vi "2D Table get 1D Rows.vi"(5 "data":string[][](array[string])) -> (2 "Rows":string[](array[string]))   [LabVIEW 2014]
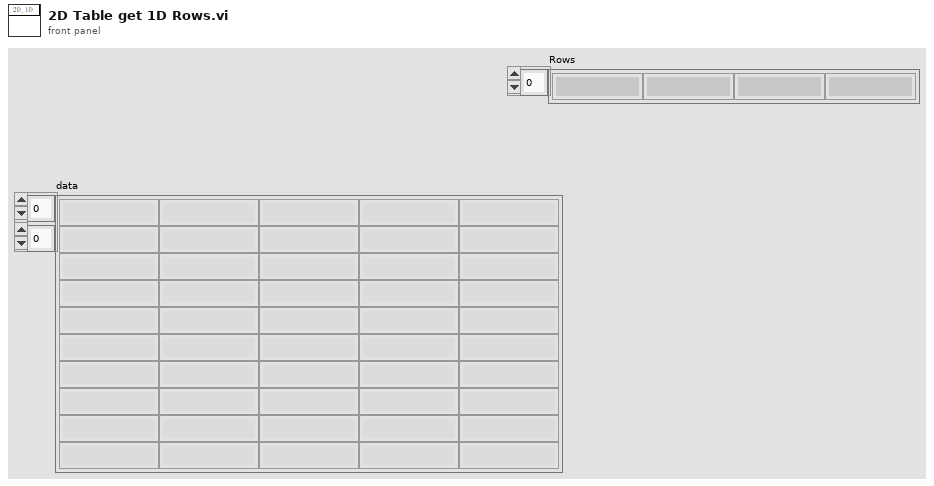
[diagram p1: front panel]
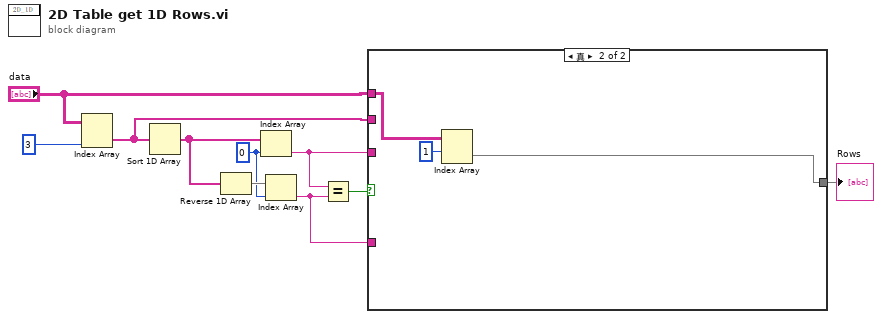
[diagram p0: block diagram]
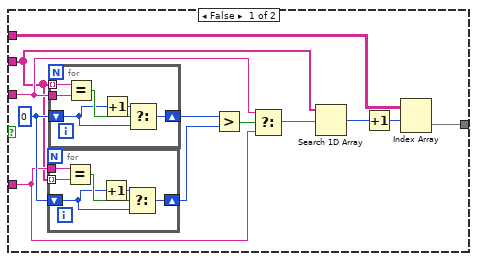
[diagram p2: hidden frame]
diagram:
  w7 = 0 ("index")
  n1 = Index Array(array="data", index (col)=3 ("disabled index (col)")) -> (element=w2:string[])  [unwired: 1 in]
  n2 = Sort 1D Array(array=w2) -> (sorted array=w9:string[])
  n3 = Reverse 1D Array(array=w9) -> (reversed array=w8:string[])
  n4 = Index Array(array=w9, index=w7) -> (element=w4:string)
  n5 = Index Array(array=w8, index=w7) -> (element=w3:string)
  n6 = Equal?(x=w4, y=w3) -> (x = y?=w6:bool)
  n7 = case shown="真" w6 {
    tunnel: "data" -> [w14 w37]
    tunnel: w4 -> [w18 _]
    tunnel: w3 -> [w17 _]
    tunnel: w2 -> [w16 _]
    tunnel: [w13 w35] -> w1
    frame False {
      w22 = 0
      n8 = for {
        tunnel: w16 -> [w28] mode=indexing
        tunnel: w17 -> [w27]
        shift-right: [w26] -> w21
        shift-left: w22 -> [w23]
        n9 = Equal?(x=w27, y=w28) -> (x = y?=w25:bool)
        n10 = Increment(x=w23) -> (x+1=w24:i32)
        n11 = Select(t=w24, s=w25, f=w23) -> (s? t:f=w26:i32)
      }
      n12 = for {
        tunnel: w18 -> [w34]
        tunnel: w16 -> [w33] mode=indexing
        shift-right: [w32] -> w20
        shift-left: w22 -> [w29]
        n13 = Equal?(x=w33, y=w34) -> (x = y?=w31:bool)
        n14 = Increment(x=w29) -> (x+1=w30:i32)
        n15 = Select(t=w30, s=w31, f=w29) -> (s? t:f=w32:i32)
      }
      n16 = Greater?(x=w20, y=w21) -> (0:w19:bool)
      n17 = Select(t=w18, s=w19, f=w17) -> (s? t:f=w15:string)
      n18 = Search 1D Array(1D array=w16, element=w15) -> (index of element=w11:i32)  [unwired: 1 in]
      n19 = Increment(x=w11) -> (x+1=w12:i32)
      n20 = Index Array(array=w14, index (row)=w12) -> (element=w13:string[])  [unwired: 1 in]
    }
    frame True {
      n21 = Index Array(array=w37, index (row)=1) -> (element=w35:string[])  [unwired: 1 in]
    }
  }
  "Rows" <- w1
